vi "Add Item.vi"(6 "New Item Indentation":i32, 8 "error in (no error)":errorcluster, 9 "Child Text":string[](array[string]), 10 "Left Cell String":string, 11 "reference":refnum<vi>) -> (0 "error out":errorcluster, 3 "reference out":refnum<vi>)   [LabVIEW 2019, in "Tree Control.lvlib"]
doc: "Add Item in a Tree Control."
uses:
  Tree Control.lvlib
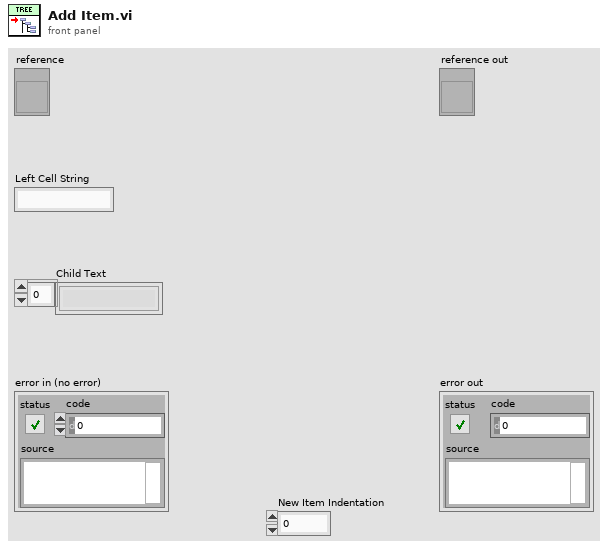
[diagram p1: front panel]
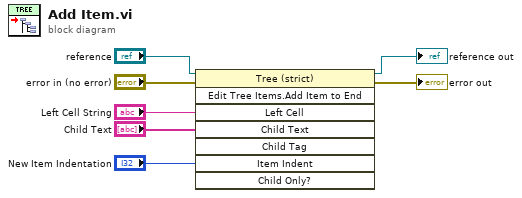
[diagram p0: block diagram]
diagram:
  n1 = invoke on="Invoke Node" class="Tree (strict)" method="Edit Tree Items.Add Item to End"(reference="reference", error in="error in (no error)", "Left Cell"="Left Cell String", "Child Text"="Child Text", "Item Indent"="New Item Indentation") -> (reference out=→"reference out":refnum<vi>, error out=→"error out":errorcluster)  [unwired: 3 in, 6 out]
